vi "find ni hardware.vi"(8 "error in (no error)":errorcluster) -> (0 "error out":errorcluster, 1 "DevNames":tag[](array[tag]), 2 "ProductType":string[](array[string]), 3 "ProductCategory":i32[](array[ring]) items=["M Series DAQ"=14643, "X Series DAQ"=15858, "E Series DAQ"=14642, "S Series DAQ"=14644, "B Series DAQ"=14662, "SC Series DAQ"=14645, "USB DAQ"=14646, "AO Series"=14647, "Digital I/O"=14648, "TIO Series"=14661, "Dynamic Signal Acquisition"=14649, "Switches"=14650, "CompactDAQ Chassis"=14658, "CompactRIO Chassis"=16144, "C Series Module"=14659, "SCXI Module"=14660, "SCC Connector Block"=14704, "SCC Module"=14705, "NI ELVIS"=14755, "Network DAQ"=14829, "SC Express"=15886, "FieldDAQ"=16151, "TestScale Chassis"=16180, "TestScale Module"=16181, "mioDAQ"=16182, "Unknown"=12588])   [LabVIEW 2025, in "Wheatstone Bridge.lvlib" / "Wheatstone Bridge.lvclass"]
uses:
  Wheatstone Bridge.lvclass
  Wheatstone Bridge.lvclass/Wheatstone Bridge.ctl
  <resource>/objmgr/daqmx.rc
panel:
  out "?":tag
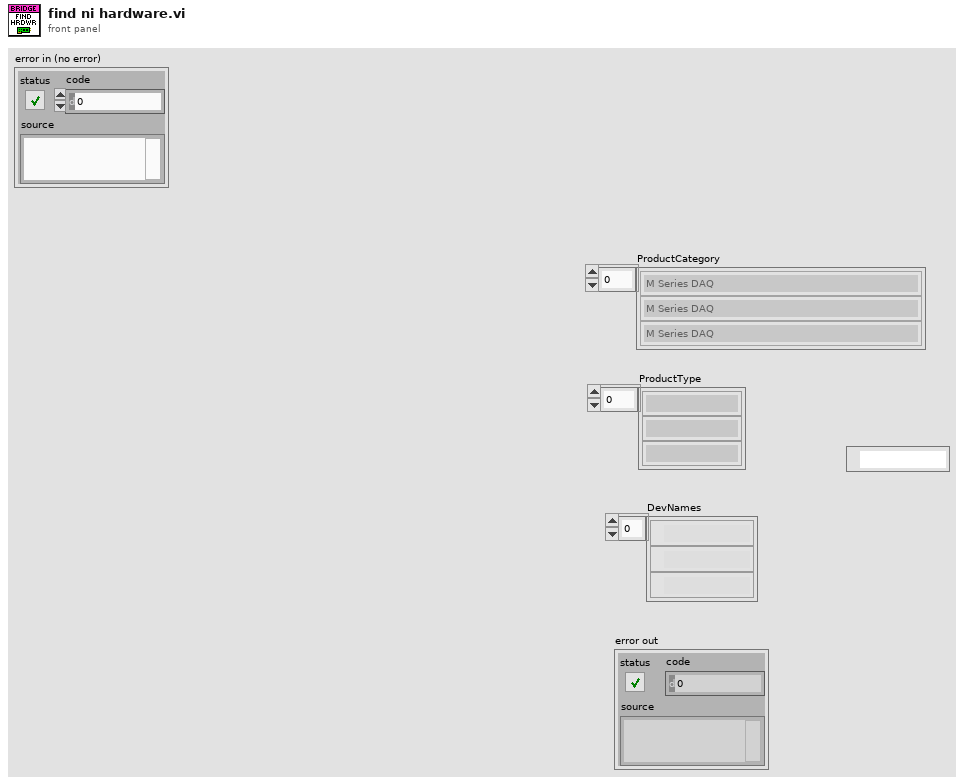
[diagram p1: front panel]
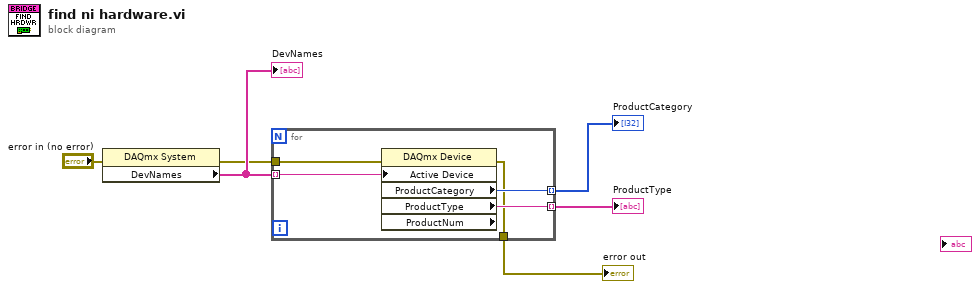
[diagram p0: block diagram]
diagram:
  n1 = property class="DAQmx System"(error in="error in (no error)") -> (error out=w1:errorcluster, "DevNames"=w6:tag[])  [unwired: 1 in, 1 out]
  "DevNames" <- w6
  n2 = for {
    tunnel: w6 -> [w11] mode=indexing
    tunnel: [w10] -> w5 mode=indexing
    tunnel: [w9] -> w4 mode=indexing
    tunnel: [w8] -> w3
    tunnel: w1 -> [w7]
    n3 = property class="DAQmx Device" props=["Active Device", "ProductCategory", "ProductType", "ProductNum"](error in=w7, "Active Device"=w11) -> (error out=w8:errorcluster, "ProductCategory"=w10:i32, "ProductType"=w9:string)  [unwired: 1 in, 2 out]
  }
  "ProductCategory" <- w5
  "ProductType" <- w4
  "error out" <- w3
